vi "MRC Ds Comms Get System Time Valid.vi"(8 "error in (no error)":errorcluster) -> (0 "error out":errorcluster, 3 "valid out":u8)   [LabVIEW 2026, in "MrcLib.lvlib"]
doc: "MRC_Status MRC_CALLCONV MRC_DsComms_GetSystemTimeValid(MRC_Bool* valid);"
uses:
  MrcLib.lvlib
  MrcLib.dll
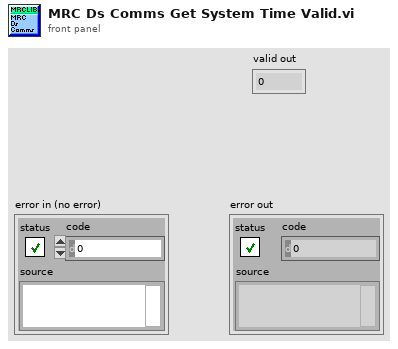
[diagram p1: front panel]
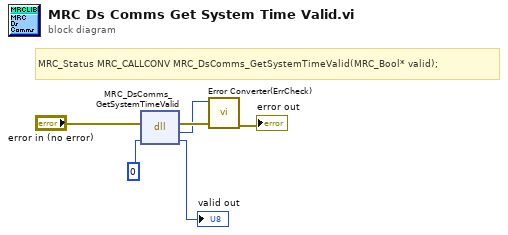
[diagram p0: block diagram]
diagram:
  # "MRC_Status MRC_CALLCONV MRC_DsComms_GetSystemTimeValid(MRC_Bool* valid);"
  n1 = dll-call lib="MrcLib.*" fn="MRC_DsComms_GetSystemTimeValid"(error in="error in (no error)", "valid"=u8 0) -> (error out=w3:errorcluster, "return type"=w1:i32, "valid"=→"valid out":u8)  [unwired: 2 in, 1 out]
  n2 = call <vilib>:"Error Converter(ErrCheck).vi"("error in (no error)"=w3, "status"=w1) -> ("error out"=→"error out":errorcluster)  [unwired: 9 in]
